vi "Read All Headers.vi"(8 "error in (no error)":errorcluster, 11 "HTTPHeaders_NET in":refnum<class "HttpHeaders_NET.lvclass">) -> (0 "error out":errorcluster, 1 "Header Values":string[](array[string]), 2 "Header Names":string[](array[string]), 3 "HTTPHeaders_NET out":refnum<class "HttpHeaders_NET.lvclass">)   [LabVIEW 2018, in "HttpClient_NET.lvlib" / "HttpHeaders_NET.lvclass"]
doc: "<b> </b> <b> </b>\nHttpClient_NET\nJustin Young - Viviota\nCopyright (c) 2021\nLicense: BSD"
uses:
  HttpHeaders_NET.lvclass
  HttpHeaders_NET.lvclass/HttpHeaders_NET.ctl
  System.Net.Http
  Accessors/Read NET_HttpHeaders.vi
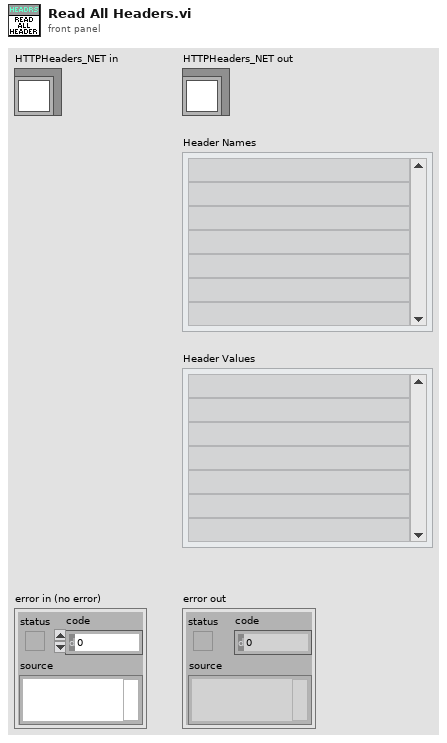
[diagram p1: front panel]
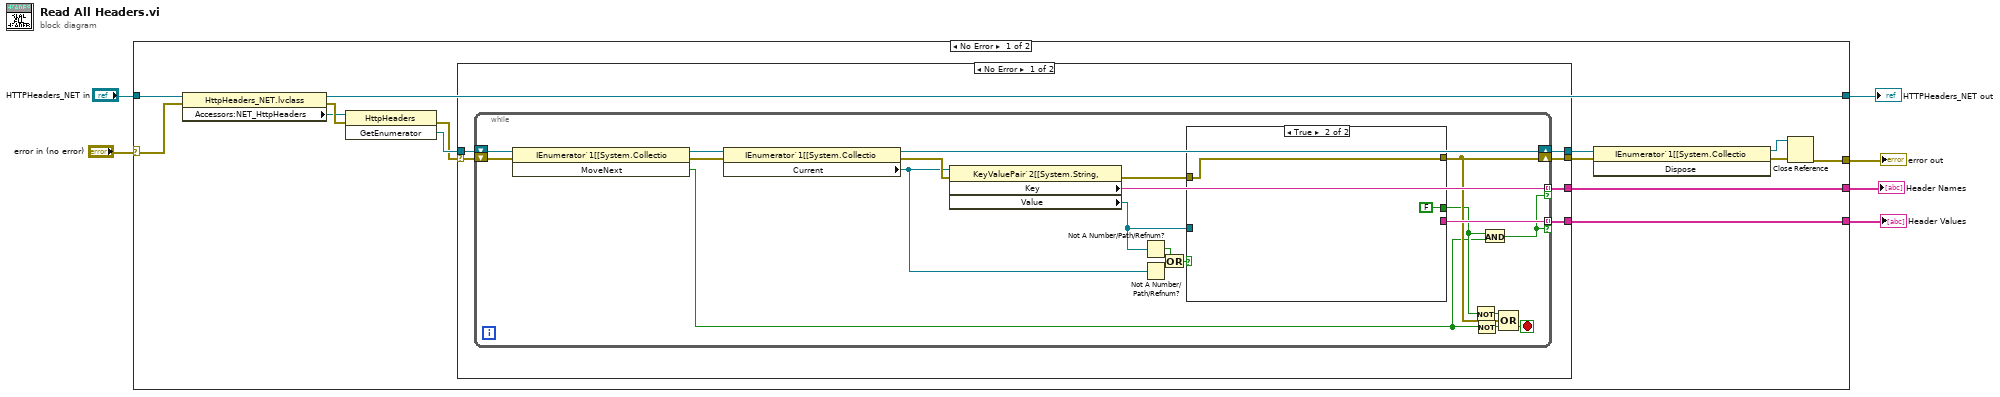
[diagram p0: block diagram]
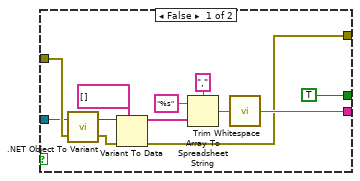
[diagram p2: hidden frame]
diagram:
  n1 = case shown="No Error" "error in (no error)" {
    selector: "error in (no error)" -> [w12 w64]
    tunnel: "HTTPHeaders_NET in" -> [w20 w65]
    tunnel: [w19 w65] -> w5
    tunnel: [w14 _] -> w4
    tunnel: [w13 _] -> w1
    tunnel: [w8 w64] -> w2
    frame No Error {
      n2 = property class="HttpHeaders_NET.lvclass"(reference=w20, error in=w12) -> (reference out=w19:refnum<class "HttpHeaders_NET.lvclass">, error out=w11:errorcluster, "Accessors:NET_HttpHeaders"=w7:refnum<k24>)
      n3 = invoke class="HttpHeaders" method="GetEnumerator"(reference=w7, error in=w11) -> (error out=w10:errorcluster, "GetEnumerator"=w16:refnum<k24>)  [unwired: 1 in, 1 out]
      n4 = case shown="No Error" w10 {
        selector: w10 -> [w22 w62]
        tunnel: w16 -> [w26 w63]
        tunnel: [w25 w63] -> w15
        tunnel: [w24 _] -> w14
        tunnel: [w23 _] -> w13
        tunnel: [w21 w62] -> w9
        frame No Error {
          n5 = while {
            shift-right: [w46] -> w25
            shift-left: w26 -> [w39]
            tunnel: [w45] -> w24 mode=indexing if=w27
            tunnel: [w44] -> w23 mode=indexing if=w27
            shift-right: [w32] -> w21
            shift-left: w22 -> [w43]
            stop <- w41 stop-if-true
            n6 = invoke class="IEnumerator`1[[System.Collectio" method="MoveNext"(reference=w39, error in=w43) -> (reference out=w47:refnum<k24>, error out=w40:errorcluster, "MoveNext"=w28:bool)  [unwired: 1 in]
            n7 = property class="IEnumerator`1[[System.Collectio"(reference=w47, error in=w40) -> (reference out=w46:refnum<k24>, error out=w42:errorcluster, "Current"=w38:refnum<k24>)
            n8 = property class="KeyValuePair`2[[System.String, "(reference=w38, error in=w42) -> (error out=w37:errorcluster, "Key"=w45:string, "Value"=w36:refnum<k24>)  [unwired: 1 out]
            n9 = Not A Number/Path/Refnum?(number/path/refnum=w36) -> (NaN/Path/Refnum?=w34:bool)
            n10 = Not A Number/Path/Refnum?(number/path/refnum=w38) -> (NaN/Path/Refnum?=w35:bool)
            n11 = Or(x=w34, y=w35) -> (x .or. y?=w33:bool)
            n12 = case shown="True" w33 {
              tunnel: [w59 _] -> w44
              tunnel: [w58 w60] -> w32
              tunnel: [TRUE FALSE] -> w29
              tunnel: w37 -> [w50 w60]
              tunnel: w36 -> [w48 _]
              frame False {
                n13 = call <vilib>:".NET Object To Variant.vi"("error in (no error)"=w50, ".NET object"=w48) -> ("error out"=w49:errorcluster, "variant"=w56:variant)
                n14 = Variant To Data(error in=w49, type=string[] [], Variant=w56) -> (data=w54:string[], error out=w58:errorcluster)
                n15 = Array To Spreadsheet String(delimiter (Tab)=",", array=w54, 3:"%s" ("format string")) -> (spreadsheet string=w51:string)
                n16 = call <vilib>:"Trim Whitespace.vi"("string"=w51) -> ("trimmed string"=w59:string)  [unwired: 1 in]
              }
              frame True {
              }
            }
            n17 = Not(x=w29) -> (.not. x?=w31:bool)
            n18 = Not(x=w28) -> (.not. x?=w30:bool)
            n19 = And(x=w29, y=w28) -> (x .and. y?=w27:bool)
            n20 = Compound Arithmetic op=OR(w31, w32, w30) -> (w41:bool)
          }
        }
        frame Error {
        }
      }
      n21 = invoke class="IEnumerator`1[[System.Collectio" method="Dispose"(reference=w15, error in=w9) -> (reference out=w17:refnum<k24>, error out=w18:errorcluster)  [unwired: 1 in, 1 out]
      n22 = Close Reference(reference=w17, error in (no error)=w18) -> (error out=w8:errorcluster)
    }
    frame Error {
    }
  }
  "error out" <- w2
  "HTTPHeaders_NET out" <- w5
  "Header Names" <- w4
  "Header Values" <- w1
